vi "Drivetrain Loop_REMOTE_13624.vi"() -> ()   [LabVIEW 2015]
uses:
  Common Code/Drivetrain Modes.ctl
  Common Code/Change Detect Boolean.vi
  Robot Global Data.vi
  <vilib>/Rock Robotics/WPI/Solenoid/Deprecated/WPI_SolenoidSetBool.vi
panel:
  in  "Reset The clocks":bool
  out "Out 4":dbl
  out "Out 3":dbl
  in  "In 4":dbl
  in  "In 3":dbl
  out "Out 2":dbl
  out "Out 1":dbl
  in  "In 2":dbl
  in  "In 1":dbl
  in  "SavedTime1":dbl
  in  "SavedTime2":dbl
  out "Modes":T1=enum."Vision Targeting"
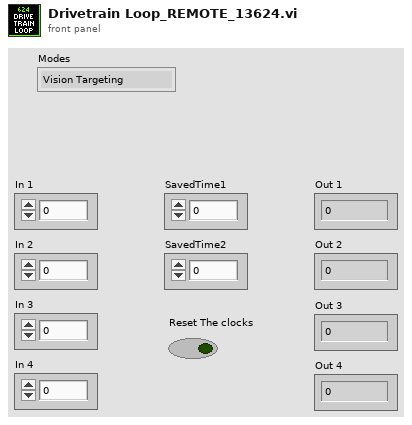
[diagram p1: front panel]
types:
  T1 = typedef "Drivetrain Modes.ctl" = enum16{"Climb", "Manual", "Vision Targeting", "PID Distance Drive", "Hybrid"}
  T2 = typedef "Drivetrain Commands.ctl" = cluster{"Y Power":dbl, "Turn Power":dbl, "1st Gear?":bool, "Modes":T1, "Heading Target":dbl, "X Max Speed":dbl, "Y Max Speed":dbl, "X Min Speed":dbl, "Y Min Speed":dbl, "Y Target":dbl}
  T3 = typedef "Dashboard Control Data.ctl" = cluster{"Shooter Presets":T4, "Encoder Control":T6, "Steer PID output":cluster{"output high":dbl, "output low":dbl}, " Steer PID gains":cluster{"proportional gain (Kc)":dbl, "integral time (Ti, min)":dbl, "derivative time (Td, min)":dbl}, "Drivetrain Settings":T7, "Vision Packet":T8, "Dashboard Drivetrain Command":T9, "Intake Command Cluster":T11}
  T4 = typedef "Shooter Presets.ctl" = cluster{"Batter Shot":T5, "Low Bar Curve Shot":T5, "Deep Middle Shot":T5, "Manual Shot":T5, "Left Ticks Per Rotation":dbl, "Right Ticks Per Rotation":dbl, "Low Bar Shot":T5, "Shooter RPM Tolerance":dbl, "IIR Filter Power":dbl, "Trigger Power":dbl, "Fire from Load Delay":i32, "Angle Pot Scale Factor":dbl, "Angle Pot Zero":dbl, "Shooter Deck Length":dbl, "String Pot Dist From Pivot":dbl, "Angle PID gains":cluster{"proportional gain (Kc)":dbl, "integral time (Ti, min)":dbl, "derivative time (Td, min)":dbl}, "Angle Motor Output Range":cluster{"output high":dbl, "output low":dbl}, "Shooter Angle Tolerance":dbl, "Axis Camera Angle":dbl}
  T5 = typedef "Shot Presets.ctl" = cluster{"Left Wheel RPM":dbl, "Right Wheel RPM":dbl, "Angle":dbl}
  T6 = typedef "Encoder Control.ctl" = cluster{"Right Tick Constant":dbl, "Left Tick Constant":dbl, "Reset?":bool, "Y Dist":cluster{"PID gains":cluster{"proportional gain (Kc)":dbl, "integral time (Ti, min)":dbl, "derivative time (Td, min)":dbl}}, "Y Stop Thresh":dbl, "Y Stop Speed":dbl}
  T7 = typedef "Drivetrain Settings.ctl" = cluster{"Gyro Tolerance":dbl, "Throttle Ramp (ms)":dbl, "Angular rate compensation":bool, "Throttle to Rate Scale":dbl, "Rate compensation gain":dbl}
  T8 = typedef "Vision Packet.ctl" = cluster{"Distance":dbl, "Center X":dbl, "Center Y":dbl, "Found Target?":bool}
  T9 = typedef "Dashboard Drivetrain Command.ctl" = cluster{"Drivetrain Vision":T10, "Vision Scale Down Speed":dbl, "Vision PID gains":cluster{"proportional gain (Kc)":dbl, "integral time (Ti, min)":dbl, "derivative time (Td, min)":dbl}}
  T10 = typedef "Drivetrain Vision.ctl" = cluster{"High parameters":dbl, "Low parameters":dbl}
  T11 = typedef "Intake Command Cluster.ctl" = cluster{"Suck Speed":dbl, "Spit Speed":dbl, "Right Pot 0":dbl, "Left Pot 0":dbl, "Trigger Power":dbl, "Raise Speed":dbl, "Lower Speed":dbl}
  T12 = typedef "WPI_SolenoidDevRef.ctl" = cluster{"DevStatus":errorcluster, "Pneumatics Control Module":u8, "Forward Solenoid Channel":T13, "Reverse Solenoid Channel":T13}
  T13 = typedef "WPI_SolenoidChannel.ctl" = enum8{"Solenoid 0", "Solenoid 1", "Solenoid 2", "Solenoid 3", "Solenoid 4", "Solenoid 5", "Solenoid 6", "Solenoid 7", "Invalid"}
  T14 = typedef "Dist Drive Status.ctl" = cluster{"Y In Range":bool, "X In Range":bool, "Gyro In Range":bool, "Y Dist":dbl, "X Dist":dbl, "Gyro":dbl}
  T15 = typedef "WPI_MotorControlDeviceRef.ctl" = cluster{"DeviceStatus":errorcluster, "Type":T16, "PWM":cluster{"PWM Channel":T17, "DeadBand":T18}, "CAN":cluster{"Device Number":u8, "Control Mode":T19, "Semaphore":T20, "Max Vout":dbl, "TalonSRX Control Mode":T21}, "Invert":bool}
  T16 = typedef "WPI_MotorControlType.ctl" = enum16{"PWM", "CAN", "CANTalonSRX"}
  T17 = typedef "FPGA_DIOPWMChannel.ctl" = enum8{"PWM 0", "PWM 1", "PWM 2", "PWM 3", "PWM 4", "PWM 5", "PWM 6", "PWM 7", "PWM 8", "PWM 9", "PWM MXP 0", "PWM MXP 1", "PWM MXP 2", "PWM MXP 3", "PWM MXP 4", "PWM MXP 5", "PWM MXP 6", "PWM MXP 7", "PWM MXP 8", "PWM MXP 9", "Invalid"}
  T18 = typedef "WPI_PWMDeadband.ctl" = cluster{"Name":string, "maxPositivePwm":i32, "minPositivePwm":i32, "centerPwm":i32, "maxNegativePwm":i32, "minNegativePwm":i32, "angularRange":u16}
  T19 = typedef "WPI_CANJaguar_ControlMode.ctl" = enum8{"Percent VBus", "Current", "Speed", "Position", "Voltage"}
  T20 = typedef "Semaphore RefNum" = refnum<k1>
  T21 = typedef "WPI_CANTalonSRX_APIControlMode.ctl" = enum8{"Percent VBus", "Speed", "Position", "Slave", "Unchanged / Invalid", "Voltage Compensation", "Current", "Motion Profile"}
  T22 = typedef "Drivetrain Status Cluster.ctl" = cluster{"Modes":T1, "Y (Throttle)":dbl, "X (Steer)":dbl, "Gyro In Range?":bool, "Distance Drive Finished?":bool, "Stop Eject Lockout":bool, "Dist Drive Status":T14, "Y Target":dbl, "Heading Target":dbl, "Vision Target Aligned?":bool, "Gear":dbl, "1st Gear Time":dbl, "2nd Gear Time":dbl, "1st Gear Shifts":dbl, "2nd Gear Shifts":dbl}
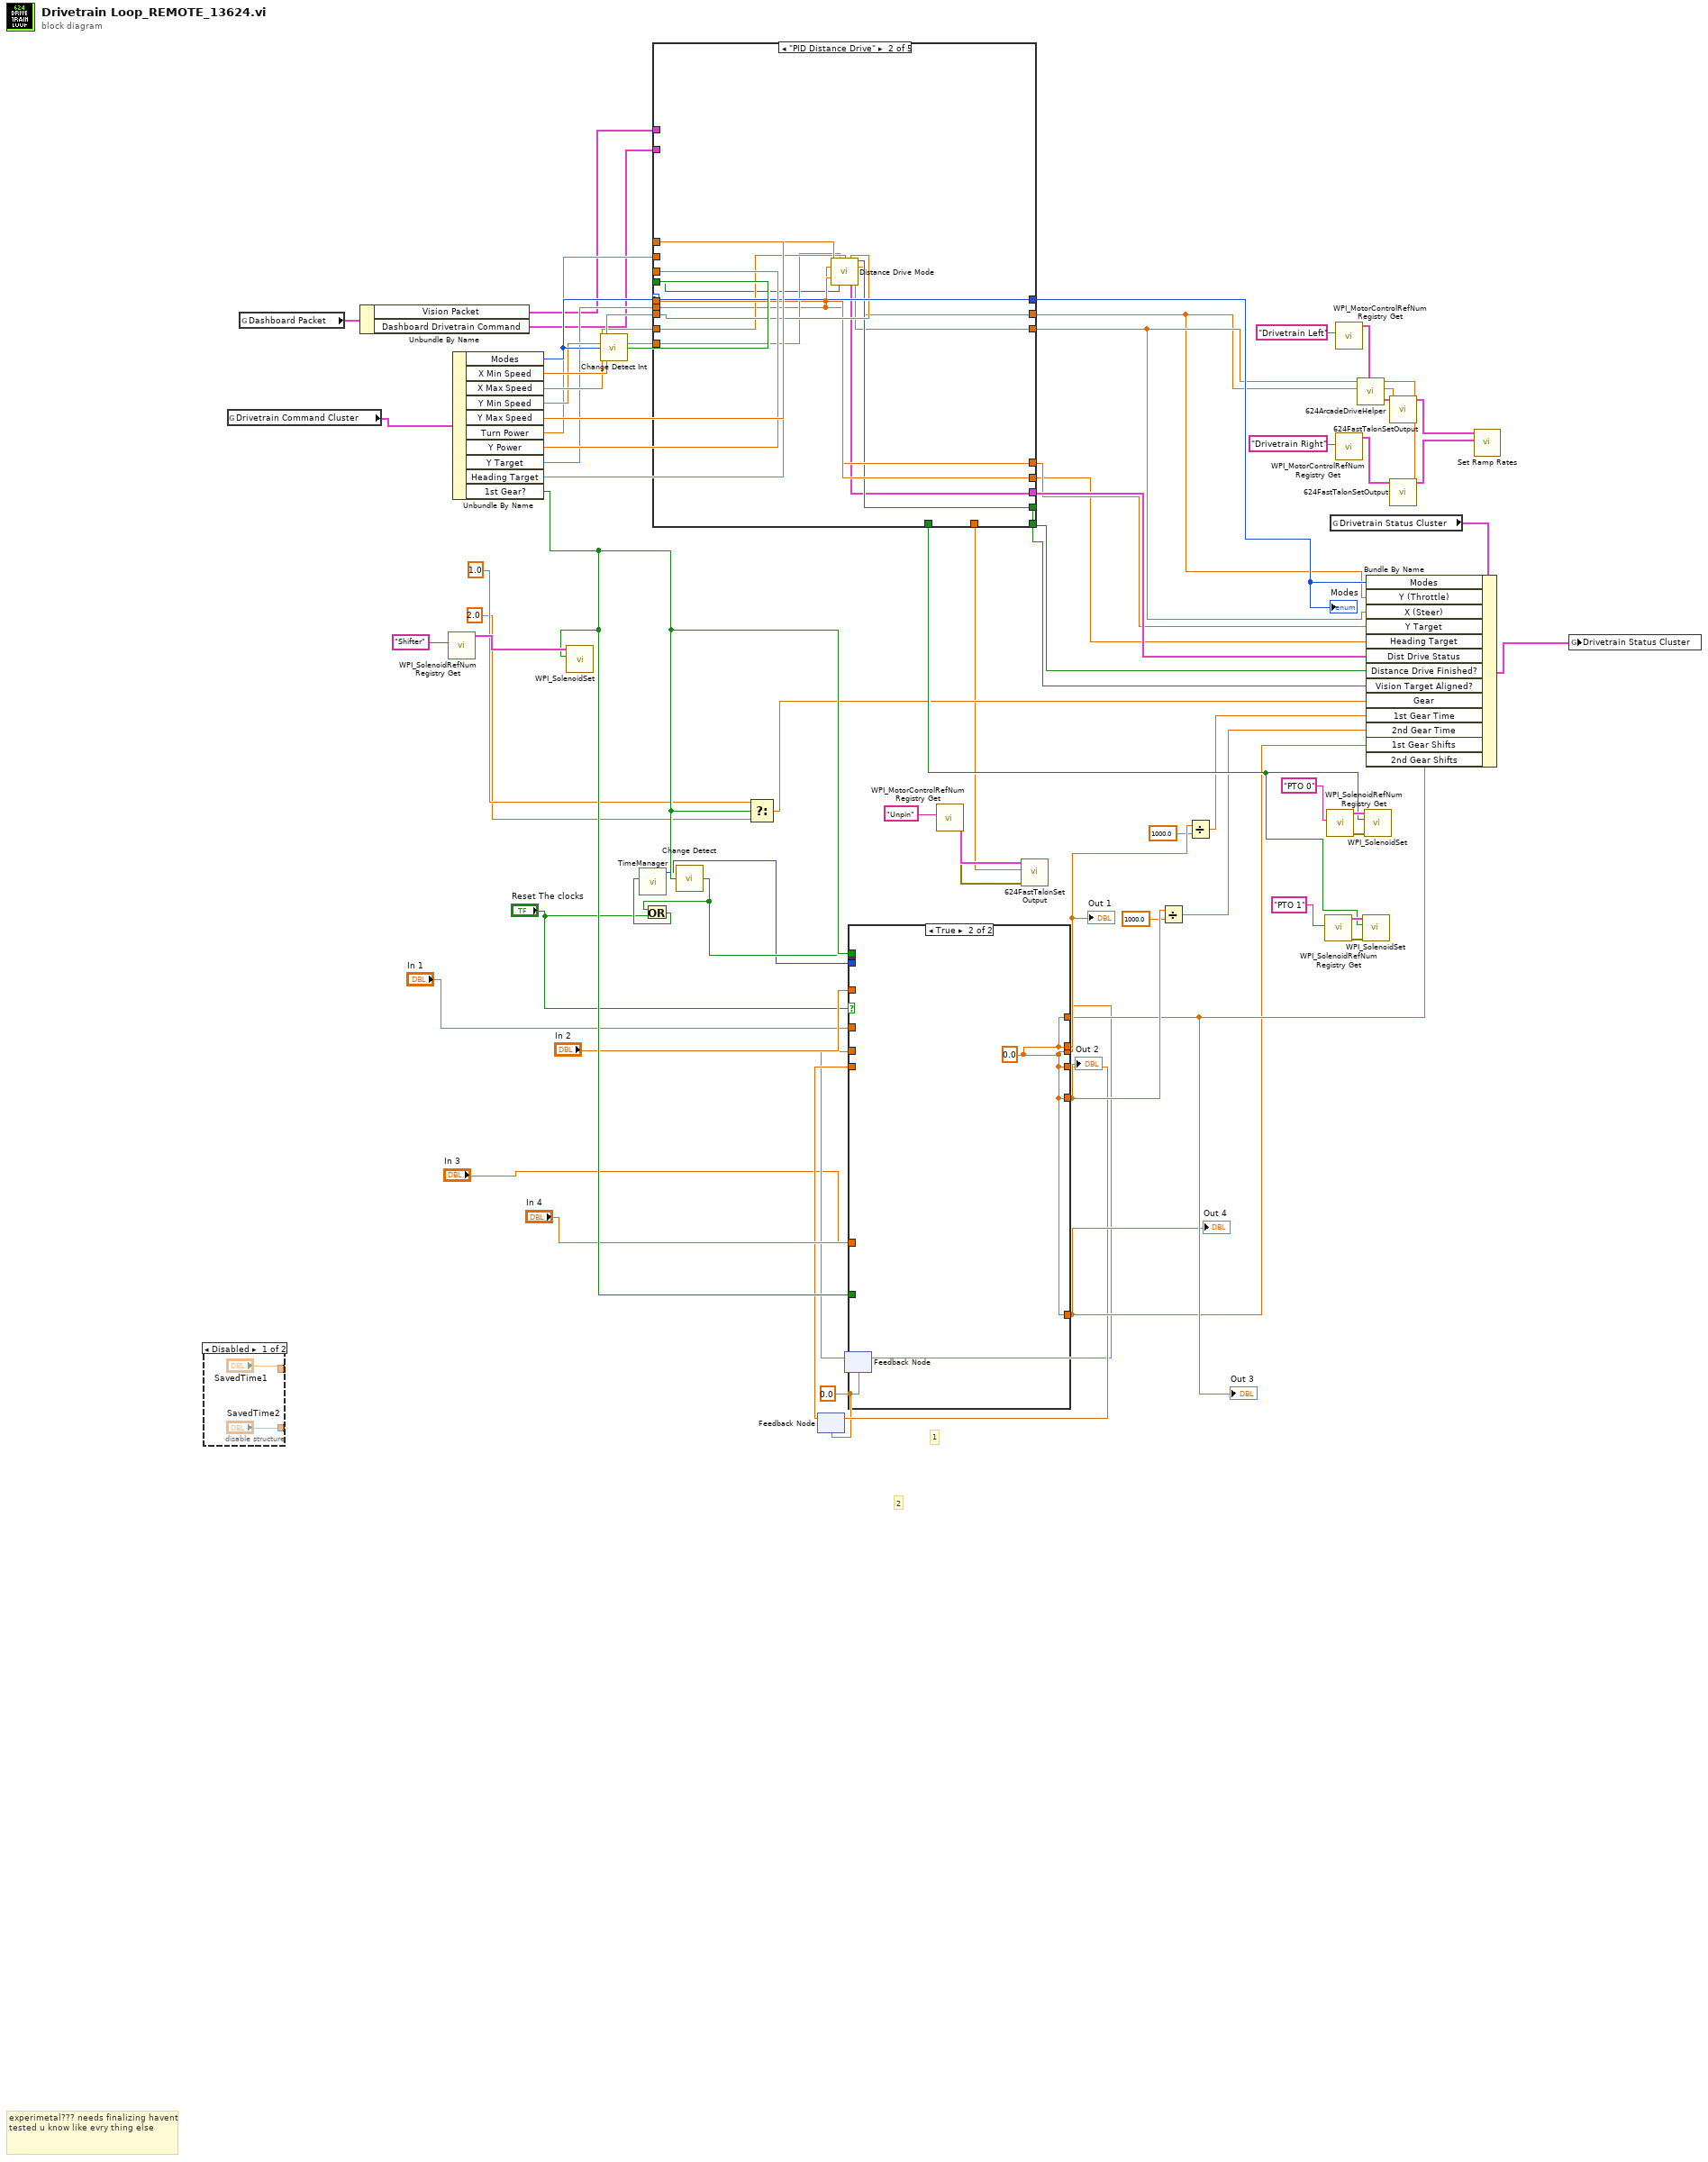
[diagram p0: block diagram]
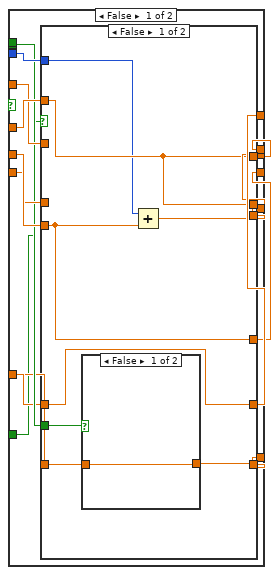
[diagram p2: hidden frame]
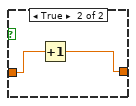
[diagram p3: hidden frame]
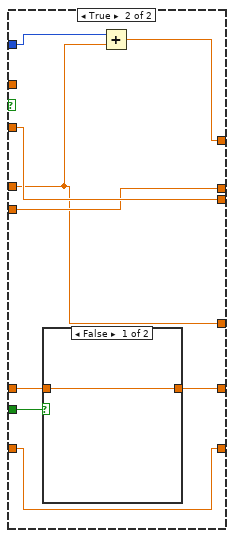
[diagram p4: hidden frame]
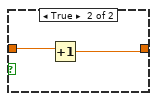
[diagram p5: hidden frame]
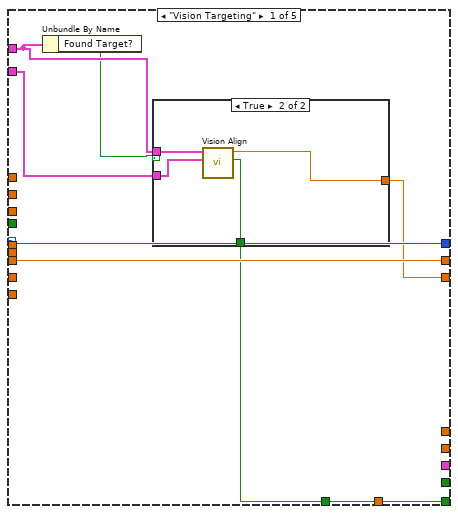
[diagram p6: hidden frame]
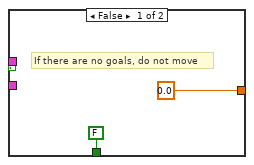
[diagram p7: hidden frame]
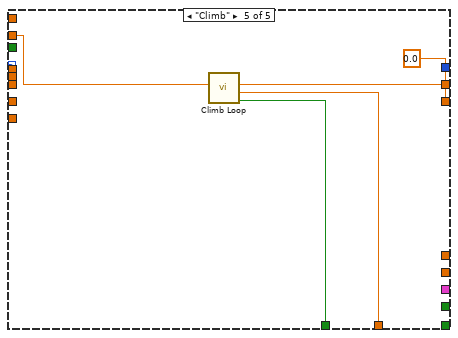
[diagram p10: hidden frame]
diagram:
  w4 = 0.0 ("In 1")
  # "1"
  # "2"
  # "experimetal??? needs finalizing havent tested u know like evry thing else"
  n1 = disable-structure shown="Disabled" {
    disable-tunnel: ["SavedTime1" _] -> _
    disable-tunnel: ["SavedTime2" _] -> _
    frame Disabled {
    }
    frame Enabled {
    }
  }
  n2 = global read "Robot Global Data.vi" "Drivetrain Command Cluster"() -> (w46:T2)
  n3 = global read "Robot Global Data.vi" "Dashboard Packet"() -> (w41:T3)
  n4 = Unbundle By Name(w41) -> ("Vision Packet"=w43:T8, "Dashboard Drivetrain Command"=w42:T9)
  n5 = call <vilib>:"WPI_SolenoidRefNum Registry Get.vi"("refnum name"="Shifter") -> ("SolenoidDevRef"=w69:T12)  [unwired: 9 in, 1 out]
  n6 = Unbundle By Name(w46) -> ("Modes"=w56:T1, "X Min Speed"=w55:dbl, "X Max Speed"=w54:dbl, "Y Min Speed"=w53:dbl, "Y Max Speed"=w52:dbl, "Turn Power"=w51:dbl, "Y Power"=w50:dbl, "Y Target"=w49:dbl, "Heading Target"=w48:dbl, "1st Gear?"=w47:bool)
  n7 = call-poly <vilib>:"WPI_SolenoidSet.vi"("Value"=w47, "SolenoidDevRef"=w69) -> ()  [unwired: 8 in, 2 out]
  n8 = call "Change Detect Int.vi"("In"=w56) -> ("Changed?"=w65:bool)
  n9 = case shown="\"PID Distance Drive\"" w56 {
    selector: w56 -> [w78 w97 _ w100 _]
    tunnel: w55 -> [w79 w96 _ _ _]
    tunnel: w54 -> [_ w94 _ _ _]
    tunnel: w53 -> [_ w93 _ _ _]
    tunnel: [w79 w88 _ w98 w101] -> w59
    tunnel: [w76 w86 _ w99 0.0] -> w60
    tunnel: [w78 w97 _ w100 _] -> w68
    tunnel: w65 -> [_ w90 _ _ _]
    tunnel: [w77 _ _ _ _] -> w19
    tunnel: [_ w87 _ _ _] -> w17
    tunnel: [_ w89 _ _ _] -> w18
    tunnel: [_ w91 _ _ _] -> w16
    tunnel: [_ w92 _ _ _] -> w15
    tunnel: w52 -> [_ w95 _ _ _]
    tunnel: w51 -> [_ _ _ w99 _]
    tunnel: w50 -> [_ _ _ w98 w104]
    tunnel: w48 -> [_ w92 _ _ _]
    tunnel: w49 -> [_ w91 _ _ _]
    tunnel: w43 -> [w75 _ _ _ _]
    tunnel: w42 -> [w73 _ _ _ _]
    tunnel: [_ _ _ _ w103] -> w33
    tunnel: [_ _ _ _ w102] -> w1
    frame "Vision Targeting" {
      n10 = Unbundle By Name(w75) -> ("Found Target?"=w74:bool)
      n11 = case shown="True" w74 {
        tunnel: [0.0 ("Turn Power") w82] -> w76
        tunnel: w73 -> [_ w85]
        tunnel: w75 -> [_ w84]
        tunnel: [FALSE ("Aligned?") w83] -> w77
        frame False {
          # "If there are no goals, do not move"
        }
        frame True {
          n12 = call "Vision Align.vi"("Dashboard Drivetrain Command"=w85, "Vision Packet"=w84) -> ("Aligned?"=w83:bool, "Turn Power"=w82:dbl)  [unwired: 8 in]
        }
      }
    }
    frame "PID Distance Drive" {
      n13 = call "Distance Drive Mode.vi"("Y Output High"=w95, "Y Output Low"=w93, "X Output High"=w94, "X Output Low"=w96, "Y target"=w91, "Heading target"=w92, "Reinitialize"=w90) -> ("isFinished"=w89:bool, "Y out"=w88:dbl, "Dist Drive Status"=w87:T14, "X out"=w86:dbl)  [unwired: 5 in]
    }
    frame "Hybrid" {
    }
    frame "Manual", Default {
    }
    frame "Climb" {
      n14 = call "Climb Loop.vi"("Y Power"=w104) -> ("Engage"=w103:bool, "Unpin"=w102:dbl, "Y Power Output"=w101:dbl)  [unwired: 8 in]
    }
  }
  "Modes" <- w68
  n15 = call-poly "Change Detect.vi"("In"=w47) -> ("Changed?"=w11:bool)
  n16 = Or(x=w11, y="Reset The clocks") -> (x .or. y?=w10:bool)
  n17 = call "TimeManager.vi"("Reset?"=w10) -> ("Time Since Reset"=w8:u32)  [unwired: 9 in, 1 out]
  n18 = Select(t=1.0, s=w47, f=2.0) -> (s? t:f=w14:dbl)
  n19 = feedback #1(w4) -> (w5:dbl)
  n20 = feedback #2(w4) -> (w3:dbl)
  n21 = case shown="True" "Reset The clocks" {
    tunnel: "In 2" -> [w119 _]
    tunnel: "In 1" -> [w120 _]
    tunnel: w11 -> [w113 _]
    tunnel: [w111 w144] -> w28
    tunnel: w5 -> [w114 _]
    tunnel: [w108 w144] -> w26
    tunnel: w3 -> [w115 _]
    tunnel: [w107 w144] -> w25
    tunnel: [w116 w144] -> w29
    tunnel: [w117 w144] -> w30
    tunnel: [w109 w144] -> w27
    tunnel: w8 -> [w118 _]
    tunnel: w47 -> [_ _]
    tunnel: w47 -> [w106 _]
    tunnel: "In 4" -> [w110 _]
    tunnel: "In 3" -> [w112 _]
    frame False {
      n22 = case shown="False" w106 {
        tunnel: w120 -> [w128 _]
        tunnel: w119 -> [_ w140]
        tunnel: w118 -> [w127 w139]
        tunnel: [w122 w140] -> w117
        tunnel: [w128 w132] -> w116
        tunnel: w115 -> [w126 w138]
        tunnel: w114 -> [_ w137]
        tunnel: w113 -> [w125 w136]
        tunnel: w112 -> [w124 w135]
        tunnel: [w124 w133] -> w111
        tunnel: w110 -> [w123 w134]
        tunnel: [w121 w134] -> w109
        tunnel: [w126 w137] -> w108
        tunnel: [w128 w138] -> w107
        frame False {
          n23 = case shown="False" w125 {
            tunnel: w123 -> [w129 w131]
            tunnel: [w129 w130] -> w121
            frame False {
            }
            frame True {
              n24 = Increment(x=w131) -> (x+1=w130:dbl)
            }
          }
          n25 = Add(x=w127, y=w126) -> (x+y=w122:dbl)
        }
        frame True {
          n26 = case shown="False" w136 {
            tunnel: w135 -> [w141 w143]
            tunnel: [w141 w142] -> w133
            frame False {
            }
            frame True {
              n27 = Increment(x=w143) -> (x+1=w142:dbl)
            }
          }
          n28 = Add(x=w139, y=w137) -> (x+y=w132:dbl)
        }
      }
    }
    frame True {
      w144 = 0.0 ("In 1")
    }
  }
  "Out 3" <- w28
  "Out 1" <- w29
  "Out 2" <- w30
  "Out 4" <- w27
  n29 = feedback-in #1(w26) -> ()
  n30 = feedback-in #2(w25) -> ()
  n31 = call <vilib>:"WPI_MotorControlRefNum Registry Get.vi"("refnum name"="Unpin") -> ("error out"=w31:errorcluster, "MotorControlDevRef"=w32:T15)  [unwired: 9 in]
  n32 = call "624FastTalonSetOutput.vi"("error in (no error)"=w31, "Output"=w1, "MotorControlDevRef"=w32) -> ()  [unwired: 7 in, 2 out]
  n33 = Divide(x=w30, y=1000.0) -> (x/y=w21:dbl)
  n34 = Divide(x=w29, y=1000.0) -> (x/y=w23:dbl)
  n35 = call <vilib>:"WPI_SolenoidRefNum Registry Get.vi"("refnum name"="PTO 1") -> ("error out"=w39:errorcluster, "SolenoidDevRef"=w38:T12)  [unwired: 9 in]
  n36 = call <vilib>:"WPI_SolenoidRefNum Registry Get.vi"("refnum name"="PTO 0") -> ("error out"=w37:errorcluster, "SolenoidDevRef"=w36:T12)  [unwired: 9 in]
  n37 = global read "Robot Global Data.vi" "Drivetrain Status Cluster"() -> (w13:T22)
  n38 = call <vilib>:"WPI_MotorControlRefNum Registry Get.vi"("refnum name"="Drivetrain Left") -> ("MotorControlDevRef"=w63:T15)  [unwired: 9 in, 1 out]
  n39 = call <vilib>:"WPI_MotorControlRefNum Registry Get.vi"("refnum name"="Drivetrain Right") -> ("MotorControlDevRef"=w64:T15)  [unwired: 9 in, 1 out]
  n40 = call "624ArcadeDriveHelper.vi"("Y Power"=w59, "Turn Power"=w60) -> ("Left"=w57:dbl, "Right"=w58:dbl)  [unwired: 8 in]
  n41 = call-poly <vilib>:"WPI_SolenoidSet.vi"("error in (no error)"=w39, "Value"=w33, "SolenoidDevRef"=w38) -> ()  [unwired: 7 in, 2 out]
  n42 = call-poly <vilib>:"WPI_SolenoidSet.vi"("error in (no error)"=w37, "Value"=w33, "SolenoidDevRef"=w36) -> ()  [unwired: 7 in, 2 out]
  n43 = Bundle By Name(cluster=w13, "Modes"=w68, "Y (Throttle)"=w59, "X (Steer)"=w60, "Y Target"=w16, "Heading Target"=w15, "Dist Drive Status"=w17, "Distance Drive Finished?"=w18, "Vision Target Aligned?"=w19, "Gear"=w14, "1st Gear Time"=w23, "2nd Gear Time"=w21, "1st Gear Shifts"=w27, "2nd Gear Shifts"=w28) -> (w24:T22)
  n44 = call "624FastTalonSetOutput.vi"("Output"=w57, "MotorControlDevRef"=w63) -> ("MotorControlDevRef"=w62:T15)  [unwired: 8 in, 1 out]
  n45 = call "624FastTalonSetOutput.vi"("Output"=w58, "MotorControlDevRef"=w64) -> ("MotorControlDevRef"=w61:T15)  [unwired: 8 in, 1 out]
  n46 = call "Set Ramp Rates.vi"("DT Right"=w61, "DT Left"=w62) -> ()  [unwired: 10 in]
  n47 = global write "Robot Global Data.vi" "Drivetrain Status Cluster"(w24) -> ()
